vi "test_FXP Signed Value Conversion_Fractional Only.vi"(8 "error in (no error)":errorcluster, 11 "TestCase in":refnum<class "FPGA Register IO Tests.lvclass">) -> (0 "error out":errorcluster, 3 "TestCase out":refnum<class "FPGA Register IO Tests.lvclass">)   [LabVIEW 2020, in "FPGA Register IO Tests.lvclass"]
uses:
  FPGA Register IO Tests.lvclass
  APIs/FPGA Register IO/TypeDefs/FXP Configuration.ctl
  <vilib>/fxp/LVFixedPointRepBitsTypeDef.ctl
  <vilib>/fxp/LVFixedPointRepRangeTypeDef.ctl
  <vilib>/addons/_JKI Toolkits/VI Tester/TestCase.llb/TestCase.lvclass
  APIs/FPGA Register IO/FPGA Register IO.lvlib
  <vilib>/Utility/Data Type/NI_Data Type.lvlib
  C:/Program Files (x86)/National Instruments/LabVIEW 2020/vi.lib/addons/_JKI Toolkits/VI Tester/TestCase.llb/TestCase.lvclass
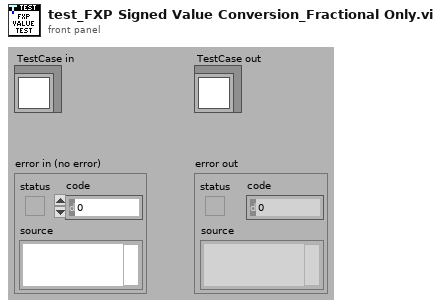
[diagram p1: front panel]
types:
  T1 = typedef "FPGA Register IO.lvlib/FXP Configuration.ctl" = cluster{"FXP Representation":T2, "FXP Range":T3}
  T2 = typedef "LVFixedPointRepBitsTypeDef.ctl" = cluster{"Signed":bool, "Word Length":u32, "Integer Word Length":i32}
  T3 = typedef "LVFixedPointRepRangeTypeDef.ctl" = cluster{"Range Min":dbl, "Range Max":dbl, "Delta":dbl}
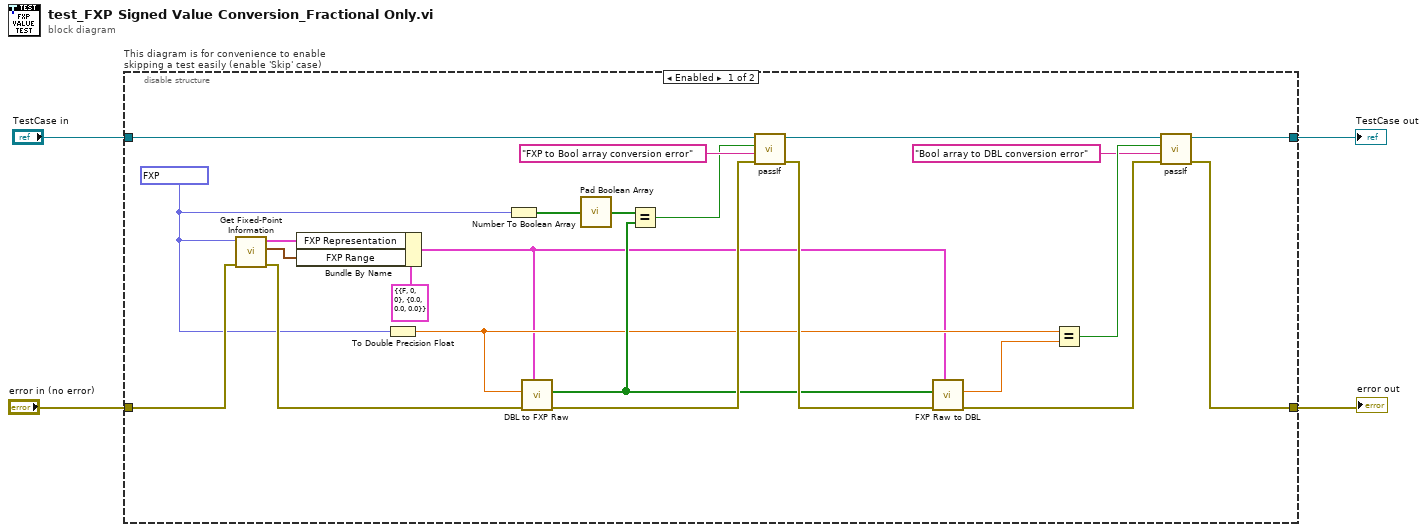
[diagram p0: block diagram]
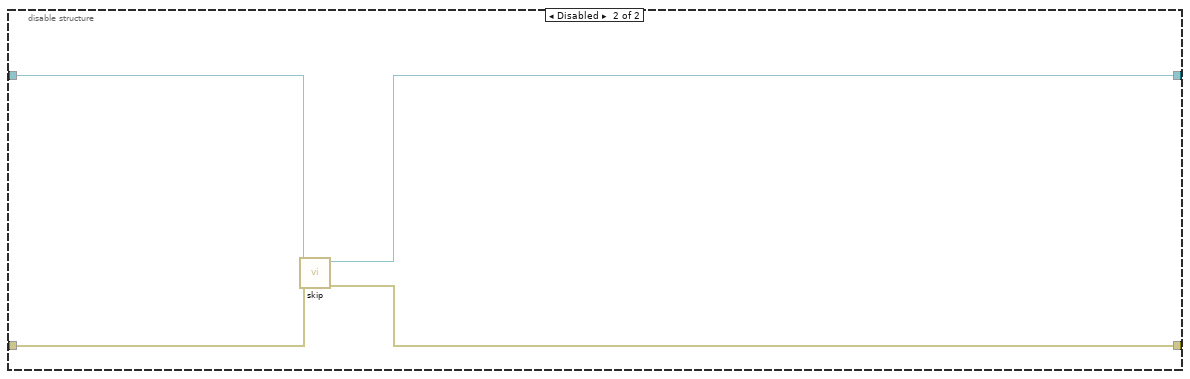
[diagram p2: hidden frame]
diagram:
  n1 = disable-structure "This diagram is for convenience to enable skipping a test easily (enable 'Skip' case)" shown="Enabled" {
    disable-tunnel: "TestCase in" -> [w27 w31]
    disable-tunnel: [w16 w29] -> w1
    disable-tunnel: [w17 w30] -> w3
    disable-tunnel: "error in (no error)" -> [w10 w28]
    frame Enabled {
      w8 = fxp<+/-,8,0> -0.30078125
      n2 = call <vilib>:"Get Fixed-Point Information.vi"("error in (no error)"=w10, "variant"=w8) -> ("error out"=w9:errorcluster, "FXP range"=w13:T3, "FXP representation"=w14:T2)  [unwired: 6 in, 1 out]
      n3 = Bundle By Name(cluster=T1 {"FXP Representation"={"Signed"=FALSE, "Word Length"=0, "Integer Word Length"=0}, "FXP Range"={"Range Min"=0.0, "Range Max"=0.0, "Delta"=0.0}} ("FXP Configuration"), "FXP Representation"=w14, "FXP Range"=w13) -> (w11:T1)
      n4 = To Double Precision Float(number=w8) -> (double precision float=w21:dbl)
      n5 = Number To Boolean Array(number=w8) -> (Boolean array=w6:bool[])
      n6 = call "DBL to FXP Raw.vi"("FXP Configuration"=w11, "error in (no error)"=w9, "DBL Value"=w21) -> ("error out"=w26:errorcluster, "Bool Data"=w23:bool[])  [unwired: 7 in]
      n7 = call "Pad Boolean Array.vi"("Boolean array in"=w6) -> ("Padded array"=w5:bool[])
      n8 = Equal?(x=w5, y=w23) -> (x = y?=w7:bool)
      n9 = call-dynamic "passIf.vi"("error in (no error)"=w26, "message (\"\")"="FXP to Bool array conversion error" ("message (\"\")"), "pass"=w7, "TestCase in"=w27) -> ("error out"=w25:errorcluster, "TestCase out"=w20:refnum<class "FPGA Register IO Tests.lvclass">)  [unwired: 6 in]
      n10 = call "FXP Raw to DBL.vi"("FXP Configuration"=w11, "error in (no error)"=w25, "Bool Data"=w23) -> ("error out"=w18:errorcluster, "DBL Value"=w22:dbl)  [unwired: 7 in]
      n11 = Equal?(x=w21, y=w22) -> (x = y?=w19:bool)
      n12 = call-dynamic "passIf.vi"("error in (no error)"=w18, "message (\"\")"="Bool array to DBL conversion error" ("message (\"\")"), "pass"=w19, "TestCase in"=w20) -> ("error out"=w17:errorcluster, "TestCase out"=w16:refnum<class "FPGA Register IO Tests.lvclass">)  [unwired: 6 in]
    }
    frame Disabled {
      # "skip test result while test is under development"
      n13 = call <vilib>:"skip.vi"("error in (no error)"=w28, "TestCase in"=w31) -> ("error out"=w30:errorcluster, "TestCase out"=w29:refnum<class "FPGA Register IO Tests.lvclass">)  [unwired: 8 in]
    }
  }
  "error out" <- w3
  "TestCase out" <- w1
